vi "Interpolate Spinner System.vi"(8 "Duration":dbl, 9 "Current Time":dbl, 10 "End SpinnerActions":T1, 11 "Start SpinnerActions":T1) -> (3 "Current SpinnerActions":T1)   [LabVIEW 2019]
uses:
  Controls/Spinner Actions.ctl
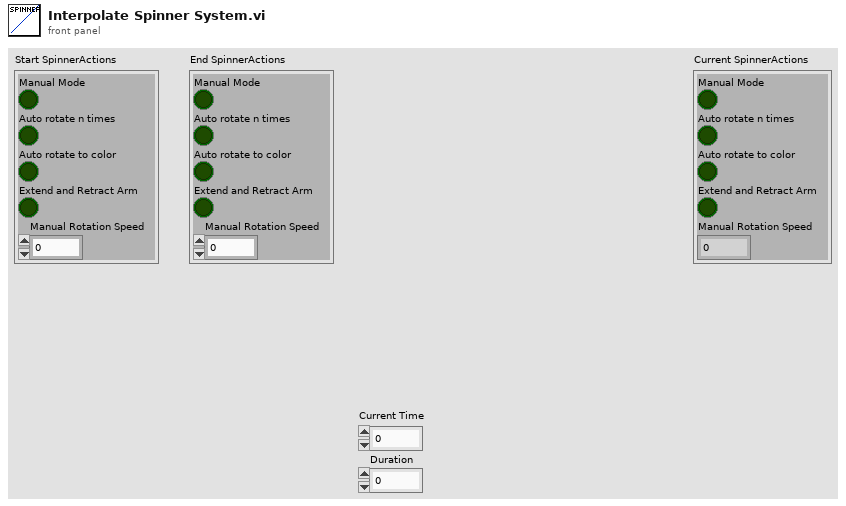
[diagram p1: front panel]
types:
  T1 = typedef "Spinner Actions.ctl" = cluster{"Manual Mode ":bool, "Auto rotate n times":bool, "Auto rotate to color\t":bool, "Extend and Retract Arm\t":bool, "Manual Rotation Speed":dbl}
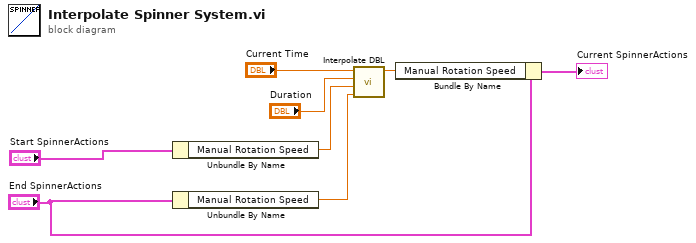
[diagram p0: block diagram]
diagram:
  n1 = Unbundle By Name("Start SpinnerActions") -> ("Manual Rotation Speed"=w8:dbl)
  n2 = Unbundle By Name("End SpinnerActions") -> ("Manual Rotation Speed"=w1:dbl)
  n3 = call "Interpolate DBL.vi"("Ending Value"=w1, "Starting Value"=w8, "Duration"="Duration", "Current Time"="Current Time") -> ("Current Value"=w7:dbl)  [unwired: 7 in]
  n4 = Bundle By Name(cluster="End SpinnerActions", "Manual Rotation Speed"=w7) -> (→"Current SpinnerActions":T1)
